vi "Macro Schema Version.vi"(8 "error in (no error)":errorcluster) -> (0 "error out":errorcluster, 3 "Macro Schema Version":string)   [LabVIEW 2023]
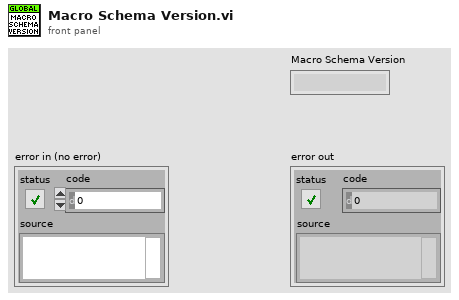
[diagram p1: front panel]
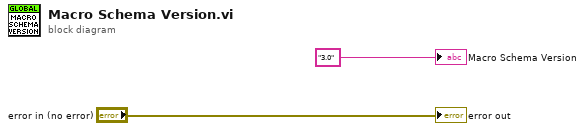
[diagram p0: block diagram]
diagram:
  "Macro Schema Version" <- "3.0" ("Macro Schema Version")
  "error out" <- "error in (no error)"
